vi "Pass If Equal 1D Array (Boolean).vi"(8 "error in (no error)":errorcluster, 9 "actual":bool[](array[boolean]), 10 "expected":bool[](array[boolean]), 11 "TestCase in":refnum<class "TestCase.lvclass">) -> (0 "error out":errorcluster, 3 "TestCase out":refnum<class "TestCase.lvclass">)   [LabVIEW 2015, in "VITAC.lvlib"]
doc: "Compares two 1D boolean arrays and returns a pass when arrays are equal.\n\nThe results string will identify the elements that don't match as well as the array index."
uses:
  VITAC.lvlib
  <vilib>/addons/_JKI Toolkits/VI Tester/TestCase.llb/TestCase.lvclass
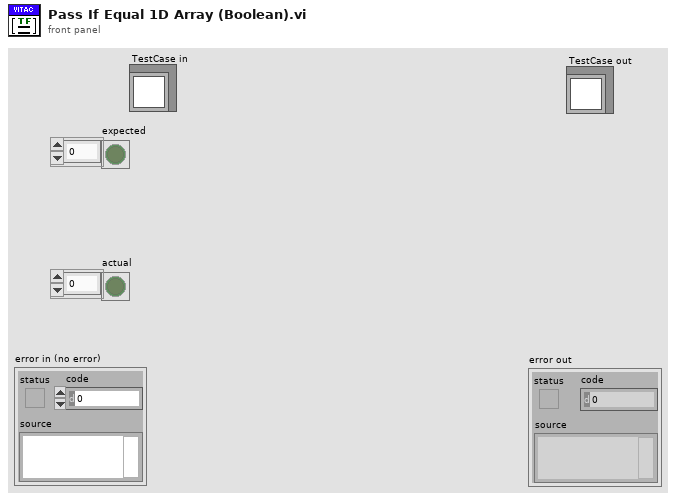
[diagram p1: front panel]
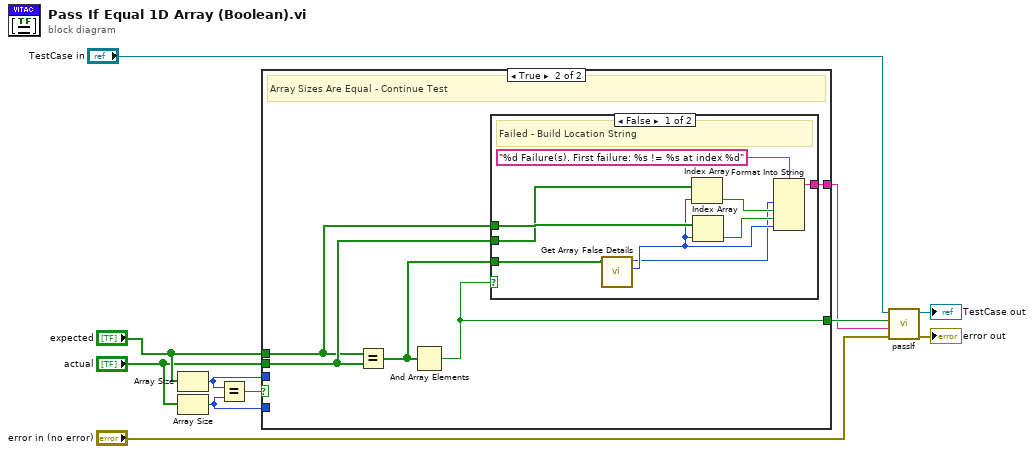
[diagram p0: block diagram]
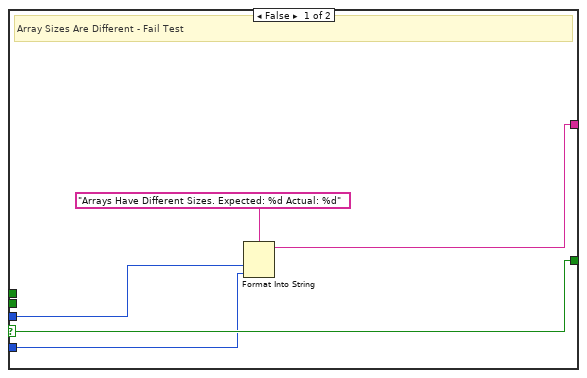
[diagram p2: hidden frame]
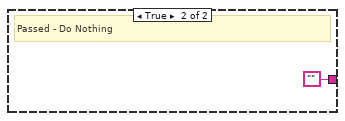
[diagram p3: hidden frame]
diagram:
  n1 = Array Size(array="expected") -> (size(s)=w2:i32)
  n2 = Array Size(array="actual") -> (size(s)=w1:i32)
  n3 = Equal?(x=w2, y=w1) -> (x = y?=w3:bool)
  n4 = case shown="True" w3 {
    selector: w3 -> [w16 _]
    tunnel: [w16 w21] -> w7
    tunnel: [w12 w20] -> w6
    tunnel: "expected" -> [_ w18]
    tunnel: "actual" -> [_ w19]
    tunnel: w2 -> [w13 _]
    tunnel: w1 -> [w14 _]
    frame False {
      # "Array Sizes Are Different - Fail Test"
      n5 = Format Into String(format string="Arrays Have Different Sizes. Expected: %d Actual: %d", w13, w14) -> (resulting string=w12:string)  [unwired: 2 in, 1 out]
    }
    frame True {
      # "Array Sizes Are Equal - Continue Test"
      n6 = Equal?(x=w18, y=w19) -> (x = y?=w17:bool[])
      n7 = And Array Elements(Boolean array=w17) -> (logical AND=w21:bool)
      n8 = case shown="False" w21 {
        tunnel: w17 -> [w24 _]
        tunnel: w18 -> [w26 _]
        tunnel: w19 -> [w25 _]
        tunnel: [w27 ""] -> w20
        frame False {
          # "Failed - Build Location String"
          n9 = call "Get Array False Details.vi"("Array"=w24) -> ("First False"=w23:i32, "Count"=w22:i16)  [unwired: 9 in]
          n10 = Index Array(array=w25, index=w23) -> (element=w29:bool)
          n11 = Index Array(array=w26, index=w23) -> (element=w28:bool)
          n12 = Format Into String(format string="%d Failure(s). First failure: %s != %s at index %d", w22, w29, w28, w23) -> (resulting string=w27:string)  [unwired: 2 in, 1 out]
        }
        frame True {
          # "Passed - Do Nothing"
        }
      }
    }
  }
  n13 = call-dynamic "passIf.vi"("error in (no error)"="error in (no error)", "message (\"\")"=w6, "pass"=w7, "TestCase in"="TestCase in") -> ("error out"=→"error out":errorcluster, "TestCase out"=→"TestCase out":refnum<class "TestCase.lvclass">)  [unwired: 6 in]
